vi "LSM9DS1_AccGyroSetup.vi"(8 "error in (no error)":errorcluster, 10 "Accel-Gyro_Settings":T1={"Accel_Range"=enum."±4g", "Gyro_Range"=enum."±500dps", "A/G_Address"=enum."0x6B", "Motion Thresh"=0.0, "reset"=FALSE}, 11 "I2C Bus":T3=enum."Invalid") -> (0 "error out":errorcluster, 1 "Gyro_Active":bool, 2 "Accel_Active":bool, 3 "I2C_A/GDevRef":T2={"DevStatus"={"status"=FALSE, "code"=0, "source"=""}, "Device Address"=0, "Handle"=0, "I2C Bus"=enum."Invalid"} {"Device Address" format="%.0x"})   [LabVIEW 2015]
uses:
  <vilib>/Rock Robotics/SystemInterfaces/i2clib/i2c_bus.ctl
  <vilib>/Rock Robotics/WPI/I2C/WPI_I2CDevRef.ctl
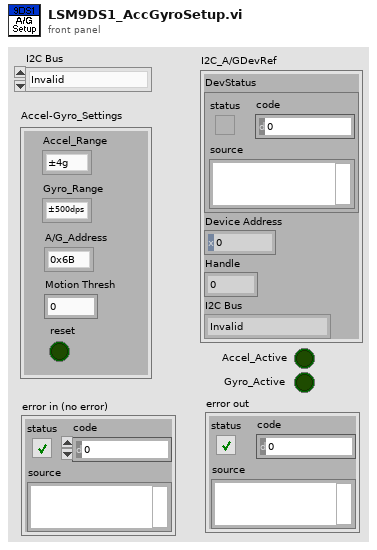
[diagram p1: front panel]
types:
  T1 = cluster{"Accel_Range":enum8{"±2g", "±16g", "±4g", "±8g", "disabled"}, "Gyro_Range":enum8{"±245dps", "±500dps", "disabled", "±2000dps"}, "A/G_Address":enum8{"0x6A", "0x6B"}, "Motion Thresh":dbl, "reset":bool}
  T2 = typedef "WPI_I2CDevRef.ctl" = cluster{"DevStatus":errorcluster, "Device Address":u8, "Handle":i32, "I2C Bus":T3}
  T3 = typedef "i2c_bus.ctl" = enum16{"I2C On-Board", "I2C MXP", "Invalid"}
  T4 = enum8{"±245dps", "±500dps", "disabled", "±2000dps"}
  T5 = cluster{"I2C Bus":T3, "Accel-Gyro_Settings":cluster{"Accel_Range":enum8{"±2g", "±16g", "±4g", "±8g", "disabled"}, "Gyro_Range":enum8{"±245dps", "±500dps", "disabled", "±2000dps"}, "A/G_Address":enum8{"0x6A", "0x6B"}, "Motion Thresh":dbl, "reset":bool}}
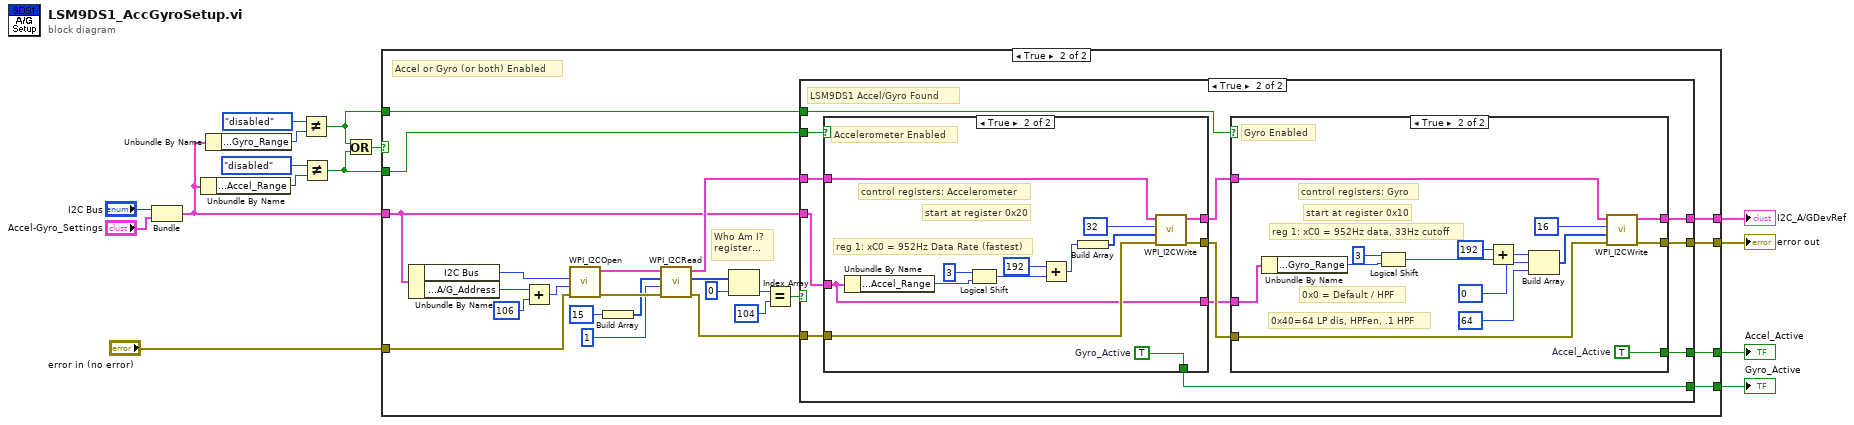
[diagram p0: block diagram]
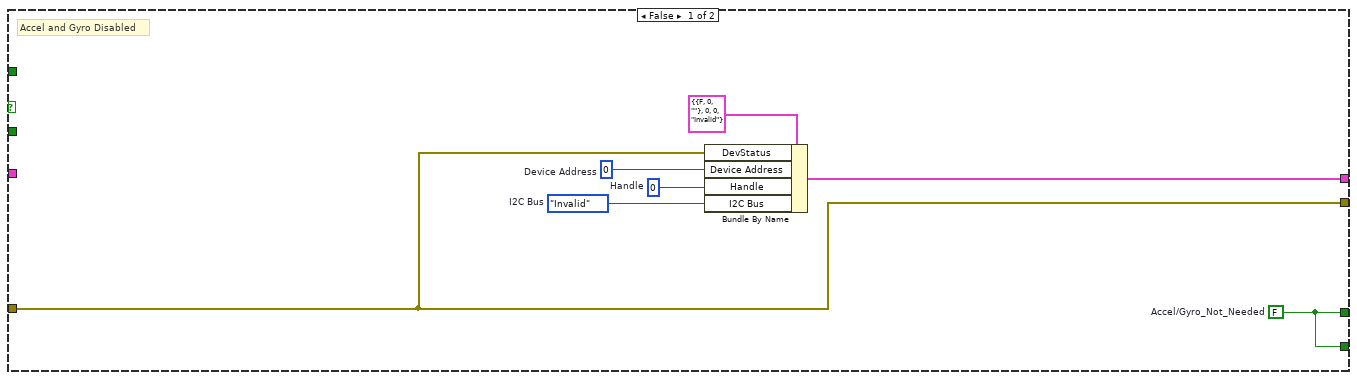
[diagram p2: hidden frame]
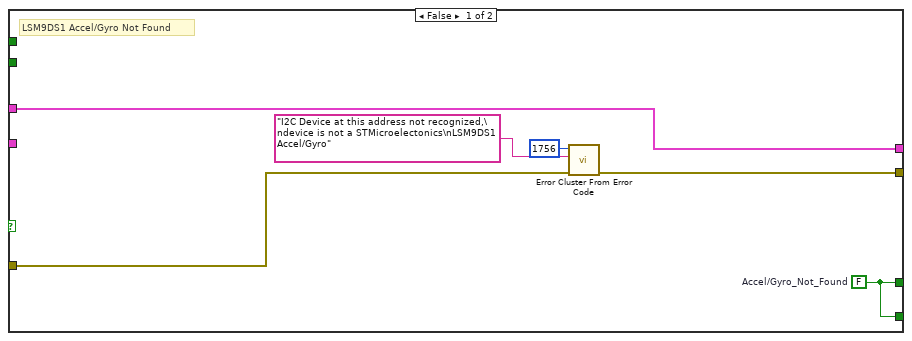
[diagram p3: hidden frame]
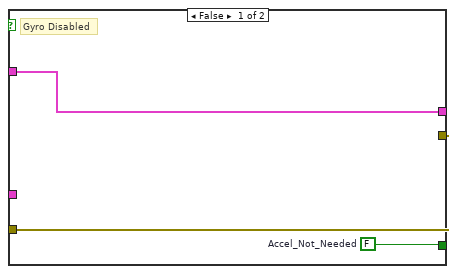
[diagram p4: hidden frame]
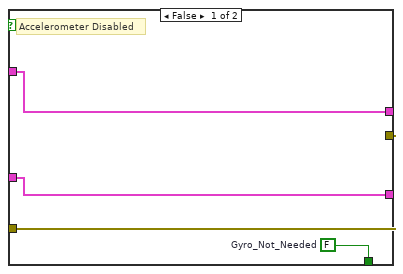
[diagram p5: hidden frame]
diagram:
  n1 = Bundle("I2C Bus"="I2C Bus", "Accel-Gyro_Settings"="Accel-Gyro_Settings") -> (w5:T5)  [unwired: 1 in]
  n2 = Unbundle By Name(w5) -> ("Accel-Gyro_Settings.Accel_Range"=w13:enum8{"±2g", "±16g", "±4g", "±8g", "disabled"})
  n3 = Unbundle By Name(w5) -> ("Accel-Gyro_Settings.Gyro_Range"=w8:T4)
  n4 = Not Equal?(x=T4."disabled" ("Gyro_Range"), y=w8) -> (x != y?=w3:bool)
  n5 = Not Equal?(x=enum8{"±2g", "±16g", "±4g", "±8g", "disabled"}."disabled" ("Accel_Range"), y=w13) -> (x != y?=w4:bool)
  n6 = Or(x=w3, y=w4) -> (x .or. y?=w6:bool)
  n7 = case shown="True" w6 {
    tunnel: "error in (no error)" -> [w17 w44]
    tunnel: w5 -> [_ w28]
    tunnel: [w17 w32] -> w12
    tunnel: [w18 w27] -> w11
    tunnel: w4 -> [_ w26]
    tunnel: w3 -> [_ w25]
    tunnel: [w16 w24] -> w2
    tunnel: [w16 w23] -> w1
    frame False {
      w16 = FALSE  # Accel/Gyro_Not_Needed
      w20 = i2c_bus."Invalid"  # I2C Bus
      w21 = 0  # Handle
      w22 = u8 0  # Device Address
      # "Accel and Gyro Disabled"
      n8 = Bundle By Name(cluster=T2 {"DevStatus"={"status"=FALSE, "code"=0, "source"=""}, "Device Address"=0, "Handle"=0, "I2C Bus"=enum."Invalid"} ("Array"), "DevStatus"=w17, "Device Address"=w22, "Handle"=w21, "I2C Bus"=w20) -> (w18:T2)
    }
    frame True {
      # "Accel or Gyro (or both) Enabled"
      # "Who Am I?\nregister..."
      n9 = Unbundle By Name(w28) -> ("I2C Bus"=w43:T3, "Accel-Gyro_Settings.A/G_Address"=w29:enum8{"0x6A", "0x6B"})
      n10 = Add ("Gyro/Accel Slave Address")(x=w29, y=u8 106) -> (x+y=w30:u8)
      n11 = call <vilib>:"WPI_I2COpen.vi"("error in"=w44, "Device Address"=w30, "I2C Bus"=w43) -> ("error out"=w41:errorcluster, "I2CDevRef"=w42:T2)  [unwired: 7 in]
      n12 = Build Array(u8 15 ("I2CRegister")) -> (w39:u8[])
      n13 = call <vilib>:"WPI_I2CRead.vi"("error in (no error)"=w41, "I2CBytesToRead"=u8 1, "I2CRegister"=w39, "I2CDevRef"=w42) -> ("error out"=w33:errorcluster, "Data Out"=w37:u8[], "I2CDevRef"=w35:T2)  [unwired: 5 in]
      n14 = Index Array(array=w37, index=0) -> (element=w45:u8)
      n15 = Equal?(x=w45, y=u8 104) -> (x = y?=w34:bool)
      n16 = case shown="True" w34 {
        tunnel: w35 -> [w48 w64]
        tunnel: w33 -> [w50 w63]
        tunnel: [w49 w58] -> w32
        tunnel: w28 -> [_ w62]
        tunnel: [w48 w59] -> w27
        tunnel: w26 -> [_ w61]
        tunnel: w25 -> [_ w56]
        tunnel: [w47 w54] -> w24
        tunnel: [w47 w53] -> w23
        frame False {
          w47 = FALSE  # Accel/Gyro_Not_Found
          # "LSM9DS1 Accel/Gyro Not Found"
          n17 = call <vilib>:"Error Cluster From Error Code.vi"("error in (no error)"=w50, "error message (\"\")"="I2C Device at this address not recognized,\ndevice is not a STMicroelectonics\nLSM9DS1 Accel/Gyro" ("error message (\"\")"), "error code (0)"=1756) -> ("error out"=w49:errorcluster)  [unwired: 6 in]
        }
        frame True {
          # "LSM9DS1 Accel/Gyro Found"
          n18 = case shown="True" w61 {
            tunnel: w64 -> [w86 w94]
            tunnel: w63 -> [w85 w93]
            tunnel: [w85 w92] -> w57
            tunnel: w62 -> [w84 w88]
            tunnel: [w86 w90] -> w60
            tunnel: [w84 w88] -> w55
            tunnel: [w83 w87] -> w54
            frame False {
              w83 = FALSE  # Gyro_Not_Needed
              # "Accelerometer Disabled"
            }
            frame True {
              w87 = TRUE  # Gyro_Active
              # "Accelerometer Enabled"
              # "reg 1: xC0 = 952Hz Data Rate (fastest)"
              # "start at register 0x20"
              # "control registers: Accelerometer"
              n19 = Unbundle By Name(w88) -> ("Accel-Gyro_Settings.Accel_Range"=w91:enum8{"±2g", "±16g", "±4g", "±8g", "disabled"})
              n20 = Logical Shift(y=u8 3, x=w91) -> (x << y=w98:u32)
              n21 = Add(x=u8 192, y=w98) -> (x+y=w89:u8)
              n22 = Build Array(w89) -> (w96:u8[])
              n23 = call <vilib>:"WPI_I2CWrite.vi"("error in (no error)"=w93, "I2CDataToSend"=w96, "I2CRegister"=u8 32 ("element"), "I2CDevRef"=w94) -> ("error out"=w92:errorcluster, "I2CDevRef"=w90:T2)  [unwired: 6 in]
            }
          }
          n24 = case shown="True" w56 {
            tunnel: w60 -> [w67 w77]
            tunnel: w57 -> [w66 w76]
            tunnel: [w66 w75] -> w58
            tunnel: [w67 w73] -> w59
            tunnel: w55 -> [_ w71]
            tunnel: [w65 w68] -> w53
            frame False {
              w65 = FALSE  # Accel_Not_Needed
              # "Gyro Disabled"
            }
            frame True {
              w68 = TRUE  # Accel_Active
              # "0x40=64 LP dis, HPFen, .1 HPF"
              # "0x0 = Default / HPF"
              # "Gyro Enabled"
              # "reg 1: xC0 = 952Hz data, 33Hz cutoff"
              # "start at register 0x10"
              # "control registers: Gyro"
              n25 = Unbundle By Name(w71) -> ("Accel-Gyro_Settings.Gyro_Range"=w74:T4)
              n26 = Logical Shift(y=u8 3, x=w74) -> (x << y=w81:u32)
              n27 = Add(x=u8 192, y=w81) -> (x+y=w72:u8)
              n28 = Build Array(w72, u8 0 ("x"), u8 64 ("element")) -> (w79:u8[])
              n29 = call <vilib>:"WPI_I2CWrite.vi"("error in (no error)"=w76, "I2CDataToSend"=w79, "I2CRegister"=u8 16 ("element"), "I2CDevRef"=w77) -> ("error out"=w75:errorcluster, "I2CDevRef"=w73:T2)  [unwired: 6 in]
            }
          }
        }
      }
    }
  }
  "error out" <- w12
  "I2C_A/GDevRef" <- w11
  "Accel_Active" <- w1
  "Gyro_Active" <- w2
